vi "EventBuilder.get library version.vi"() -> (0 "nameAndVersion":string)   [LabVIEW 2014, in "EventBuilder.lvlib"]
doc: "obtain name and version of a library as a string"
uses:
  EventBuilder.lvlib
  CSlibraries/UtilityLib/UtilityLib.lvlib
  DataLib/DataLib.lvlib
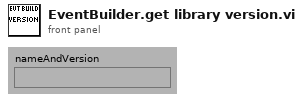
[diagram p1: front panel]
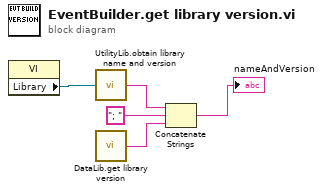
[diagram p0: block diagram]
diagram:
  n1 = property class="VI"() -> ("Library"=w5:refnum<vi>)  [unwired: 2 in, 2 out]
  n2 = call "UtilityLib.obtain library name and version.vi"("Library"=w5) -> ("nameAndVersion"=w3:string)
  n3 = call "DataLib.get library version.vi"() -> ("nameAndVersion"=w4:string)  [unwired: 1 in]
  n4 = Concatenate Strings(w3, "; " ("string"), w4) -> (→"nameAndVersion":string)
